vi "Atomic Check.VI"(1 "string":string) -> (0 "atomic":bool)   [LabVIEW 2010, in "NI_Gmath.lvlib"]
uses:
  NI_Gmath.lvlib
panel:
  # "not atomic"
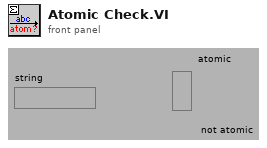
[diagram p1: front panel]
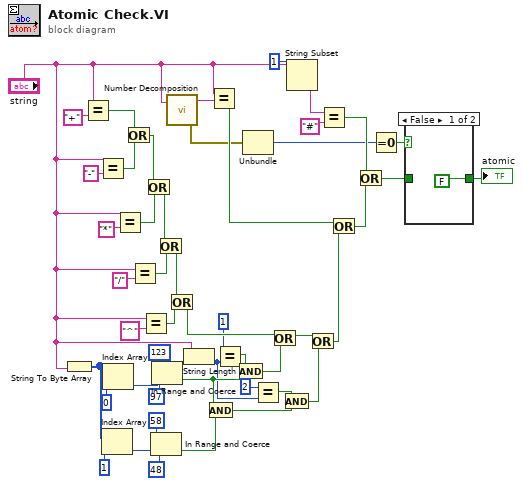
[diagram p0: block diagram]
diagram:
  n1 = String To Byte Array(string="string") -> (unsigned byte array=w16:u8[])
  n2 = Equal?(x="string", y="+") -> (x = y?=w43:bool)
  n3 = Equal?(x="string", y="-") -> (x = y?=w42:bool)
  n4 = Index Array(array=w16, index=1) -> (element=w14:u8)
  n5 = Index Array(array=w16, index=0) -> (element=w19:u8)
  n6 = Equal?(x="string", y="*") -> (x = y?=w41:bool)
  n7 = Or(x=w43, y=w42) -> (x .or. y?=w40:bool)
  n8 = Equal?(x="string", y="/") -> (x = y?=w39:bool)
  n9 = Equal?(x="string", y="^") -> (x = y?=w36:bool)
  n10 = Or(x=w40, y=w41) -> (x .or. y?=w38:bool)
  n11 = In Range and Coerce(upper limit=58, x=w14, lower limit=48) -> (In Range?=w11:bool)  [unwired: 1 out]
  n12 = In Range and Coerce(upper limit=123, x=w19, lower limit=97) -> (In Range?=w10:bool)  [unwired: 1 out]
  n13 = Or(x=w38, y=w39) -> (x .or. y?=w37:bool)
  n14 = call "Number Decomposition.VI"("number string"="string") -> ("number"=w29:string, "error out"=w2:errorcluster)  [unwired: 1 in, 1 out]
  n15 = Or(x=w37, y=w36) -> (x .or. y?=w35:bool)
  n16 = String Length(string="string") -> (length=w4:i32)
  n17 = And(x=w10, y=w11) -> (x .and. y?=w9:bool)
  n18 = Equal?(x="string", y=w29) -> (x = y?=w28:bool)
  n19 = Equal?(x=1, y=w4) -> (x = y?=w6:bool)
  n20 = And(x=w6, y=w10) -> (x .and. y?=w18:bool)
  n21 = Unbundle(w2) -> ("code"=w1:i32)  [unwired: 2 out]
  n22 = Equal?(x=2, y=w4) -> (x = y?=w3:bool)
  n23 = Or(x=w35, y=w18) -> (x .or. y?=w27:bool)
  n24 = And(x=w3, y=w9) -> (x .and. y?=w8:bool)
  n25 = String Subset(string="string", length (rest)=1) -> (substring=w33:string)  [unwired: 1 in]
  n26 = Or(x=w27, y=w8) -> (x .or. y?=w26:bool)
  n27 = Equal?(x=w33, y="#") -> (x = y?=w30:bool)
  n28 = Or(x=w28, y=w26) -> (x .or. y?=w31:bool)
  n29 = Or(x=w30, y=w31) -> (x .or. y?=w24:bool)
  n30 = Equal To 0?(x=w1) -> (x = 0?=w25:bool)
  n31 = case shown="False" w25 {
    tunnel: w24 -> [_ w50]
    tunnel: [FALSE w50] -> w23
    frame False {
    }
    frame True {
    }
  }
  "atomic" <- w23
